vi "FT_Reset_Device2011.vi"(1 "Handle":u64) -> (0 "FT_Status":u64(ring) items=["FT_OK", "FT_INVALID_HANDLE", "FT_DEVICE_NOT_FOUND", "FT_DEVICE_NOT_OPENED", "FT_IO_ERROR", "FT_INSUFFICIENT_RESOURCES", "FT_INVALID_PARAMETER", "FT_INVALID_BAUD_RATE", "FT_DEVICE_NOT_OPENED_FOR_ERASE", "FT_DEVICE_NOT_OPENED_FOR_WRITE", "FT_FAILED_TO_WRITE_DEVICE", "FT_EEPROM_READ_FAILED", "FT_EEPROM_WRITE_FAILED", "FT_EEPROM_ERASE_FAILED", "FT_EEPROM_NOT_PRESENT", "FT_EEPROM_NOT_PROGRAMMED", "FT_INVALID_ARGS", "FT_NOT_SUPPORTED", "FT_OTHER_ERROR"])   [LabVIEW 2018]
uses:
  Windows/System32/DriverStore/FileRepository/ftdibus.inf_amd64_49b3e24305b20ada/amd64/ftd2xx64.dll
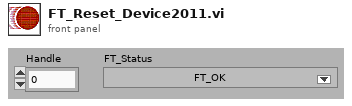
[diagram p1: front panel]
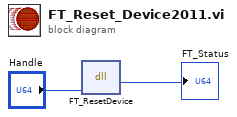
[diagram p0: block diagram]
diagram:
  n1 = dll-call lib="C:/Windows/System32/DriverStore/FileRepository/ftdibus.inf_amd64_49b3e24305b20ada/amd64/ftd2xx64.dll" fn="FT_ResetDevice"("Handle"="Handle") -> ("FT_Status"=→"FT_Status":u64)  [unwired: 4 in, 2 out]
